vi "Check OPC.vi"(8 "error in (no error)":errorcluster, 11 "OPC Queue":refnum<queue>) -> (3 "Message":string)   [LabVIEW 2020]
uses:
  support/Message Queue/Message Cluster.ctl
  support/Message Queue/Enqueue Message (Single).vi
  support/Message Queue/Message Queue.lvlib
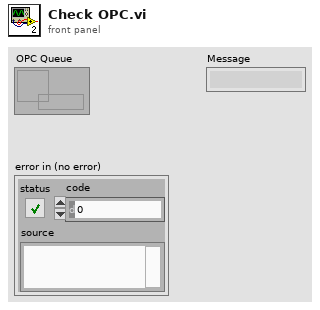
[diagram p1: front panel]
types:
  T1 = cluster{"Writer Queue":refnum<queue>, "Timeout":dbl}
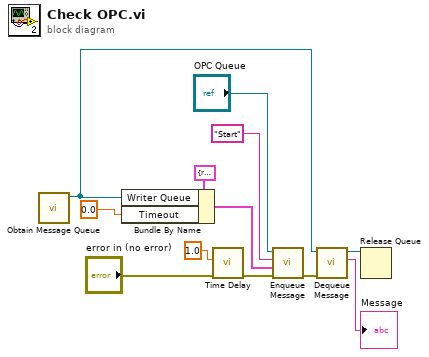
[diagram p0: block diagram]
diagram:
  n1 = call "Obtain Message Queue.vi"() -> ("Message Queue"=w8:refnum<queue>)  [unwired: 10 in, 1 out]
  n2 = Bundle By Name(cluster=T1 {"Writer Queue"=refnum, "Timeout"=0.0}, "Writer Queue"=w8, "Timeout"=0.0) -> (w5:T1)
  n3 = call "Time Delay"("error in (no error)"="error in (no error)", "Delay Time (s)"=1.0) -> ("error out"=w11:errorcluster)  [unwired: 9 in]
  n4 = call-poly "Enqueue Message.vi"("error in (no error)"=w11, "Message Data"=w5, "Message"="Start", "Message Queue"="OPC Queue") -> ("error out"=w7:errorcluster)  [unwired: 6 in, 1 out]
  n5 = call "Dequeue Message.vi"("error in (no error)"=w7, "Message Queue"=w8) -> ("Message"=→"Message":string, "dup Message Queue"=w9:refnum<queue>)  [unwired: 6 in, 2 out]
  n6 = Release Queue(queue=w9) -> ()  [unwired: 2 in, 3 out]
